vi "WLAN Tx Test Limits USL CarrierLeakage.vi"(8 "error in (no error)":errorcluster, 10 "Limits":T1 {"OBW"."Stop Frequency (Hz)" format="%#_4p"; "OBW"."Start Frequency (Hz)" format="%#_4p"; "OBW"."OBW (Hz)" format="%#_4p"}, 11 "WLAN Tx Test in":refnum<class "niDTS WLAN Tx Test.lvclass">) -> (0 "error out":errorcluster, 2 "Limits Out":T1 {"OBW"."Stop Frequency (Hz)" format="%#_4p"; "OBW"."Start Frequency (Hz)" format="%#_4p"; "OBW"."OBW (Hz)" format="%#_4p"}, 3 "WLAN Tx Test out":refnum<class "niDTS WLAN Tx Test.lvclass">)   [LabVIEW 2015, in "niDTS WLAN.lvlib" / "niDTS WLAN Tx Test.lvclass"]
uses:
  niDTS WLAN Tx Test.lvclass
  Includes/niDTS WLAN Tx Test INC Results.ctl
  Includes/niDTS WLAN Tx Test INC MOD EVM Results.ctl
  Includes/Results/niDTS Tx RES INC EVM.ctl
  Includes/niDTS WLAN Tx Test INC TXP Results.ctl
  Includes/niDTS WLAN Tx Test INC TXP Result SINGLE.ctl
  Includes/niDTS WLAN Tx Test INC OBW Results.ctl
  Instrument/INSTR TX/Results/niDTS WLAN INSTR TX INC SEM Results.ctl
  Instrument/INSTR TX/Results/niDTS WLAN INSTR TX INC SEM FSEGemts Results.ctl
  Includes/Results/niDTS Tx RES INC SEM FSEGemts.ctl
  Instrument/INSTR TX/Results/niDTS WLAN INSTR TX INC SEM MARGin Results.ctl
  Includes/Results/niDTS Tx RES INC SEM Margin.ctl
  Instrument/INSTR TX/Results/niDTS WLAN INSTR TX INC OFDM Impairments Results.ctl
  niDTS WLAN Tx Test.lvclass/niDTS WLAN Tx Test.ctl
  niDTS WLAN.lvlib
  Instrument/INSTR TX/niDTS WLAN INSTR TX.lvclass
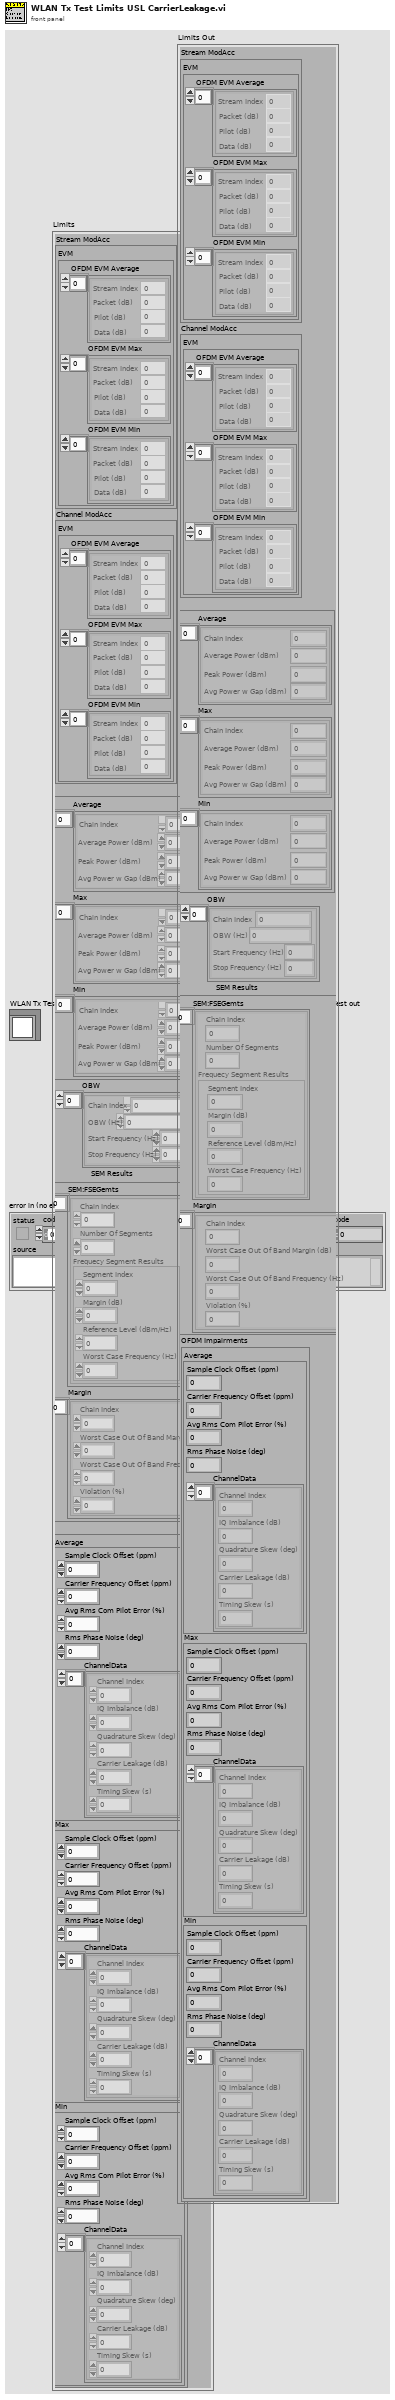
[diagram p1: front panel]
types:
  T1 = typedef "niDTS WLAN.lvlib/niDTS WLAN Tx Test INC Results.ctl" = cluster{"Stream ModAcc":T2, "Channel ModAcc":T2, "TXP":T4, "OBW":T6[], "SEM Results":T7, "OFDM Impairments":T12}
  T2 = typedef "niDTS WLAN.lvlib/niDTS WLAN Tx Test INC MOD EVM Results.ctl" = cluster{"EVM":cluster{"OFDM EVM Average":T3[], "OFDM EVM Max":T3[], "OFDM EVM Min":T3[]}}
  T3 = typedef "niDTS WLAN.lvlib/niDTS Tx RES INC EVM.ctl" = cluster{"Stream Index":i32, "Packet (dB)":dbl, "Pilot (dB)":dbl, "Data (dB)":dbl}
  T4 = typedef "niDTS WLAN.lvlib/niDTS WLAN Tx Test INC TXP Results.ctl" = cluster{"Average":T5[], "Max":T5[], "Min":T5[]}
  T5 = typedef "niDTS WLAN.lvlib/niDTS WLAN Tx Test INC TXP Result SINGLE.ctl" = cluster{"Chain Index":dbl, "Average Power (dBm)":dbl, "Peak Power (dBm)":dbl, "Avg Power w Gap (dBm)":dbl}
  T6 = typedef "niDTS WLAN.lvlib/niDTS WLAN Tx Test INC OBW Results.ctl" = cluster{"Chain Index":dbl, "OBW (Hz)":dbl, "Start Frequency (Hz)":dbl, "Stop Frequency (Hz)":dbl}
  T7 = typedef "niDTS WLAN.lvlib/niDTS WLAN INSTR TX.lvclass/niDTS WLAN INSTR TX INC SEM Results.ctl" = cluster{"SEM:FSEGemts":T8, "Margin":T10}
  T8 = typedef "niDTS WLAN.lvlib/niDTS WLAN INSTR TX.lvclass/niDTS WLAN INSTR TX INC SEM FSEGemts Results.ctl" = T9[]
  T9 = typedef "niDTS WLAN.lvlib/niDTS Tx RES INC SEM FSEGemts.ctl" = cluster{"Chain Index":i32, "Number Of Segments":i32, "Frequecy Segment Results":cluster{"Segment Index":i32, "Margin (dB)":dbl, "Reference Level (dBm/Hz)":dbl, "Worst Case Frequency (Hz)":dbl}}
  T10 = typedef "niDTS WLAN.lvlib/niDTS WLAN INSTR TX.lvclass/niDTS WLAN INSTR TX INC SEM MARGin Results.ctl" = T11[]
  T11 = typedef "niDTS WLAN.lvlib/niDTS Tx RES INC SEM Margin.ctl" = cluster{"Chain Index":i32, "Worst Case Out Of Band Margin (dB)":dbl, "Worst Case Out Of Band Frequency (Hz)":dbl, "Violation (%)":dbl}
  T12 = typedef "niDTS WLAN.lvlib/niDTS WLAN INSTR TX.lvclass/niDTS WLAN INSTR TX INC OFDM Impairments Results.ctl" = cluster{"Average":cluster{"Sample Clock Offset (ppm)":dbl, "Carrier Frequency Offset (ppm)":dbl, "Avg Rms Com Pilot Error (%)":dbl, "Rms Phase Noise (deg)":dbl, "ChannelData":cluster{"Channel Index":i32, "IQ Imbalance (dB)":dbl, "Quadrature Skew (deg)":dbl, "Carrier Leakage (dB)":dbl, "Timing Skew (s)":dbl}[]}, "Max":cluster{"Sample Clock Offset (ppm)":dbl, "Carrier Frequency Offset (ppm)":dbl, "Avg Rms Com Pilot Error (%)":dbl, "Rms Phase Noise (deg)":dbl, "ChannelData":cluster{"Channel Index":i32, "IQ Imbalance (dB)":dbl, "Quadrature Skew (deg)":dbl, "Carrier Leakage (dB)":dbl, "Timing Skew (s)":dbl}[]}, "Min":cluster{"Sample Clock Offset (ppm)":dbl, "Carrier Frequency Offset (ppm)":dbl, "Avg Rms Com Pilot Error (%)":dbl, "Rms Phase Noise (deg)":dbl, "ChannelData":cluster{"Channel Index":i32, "IQ Imbalance (dB)":dbl, "Quadrature Skew (deg)":dbl, "Carrier Leakage (dB)":dbl, "Timing Skew (s)":dbl}[]}}
  T13 = typedef "niDTS WLAN.lvlib/niDTS WLAN INC Standard.ctl" = enum16{"802.11 b DSSS", "802.11 a/g OFDM", "802.11 n HT", "802.11 ac VHT"}
  T14 = cluster{"Channel Index":i32, "IQ Imbalance (dB)":dbl, "Quadrature Skew (deg)":dbl, "Carrier Leakage (dB)":dbl, "Timing Skew (s)":dbl}[]
  T15 = cluster{"Channel Index":i32, "IQ Imbalance (dB)":dbl, "Quadrature Skew (deg)":dbl, "Carrier Leakage (dB)":dbl, "Timing Skew (s)":dbl}
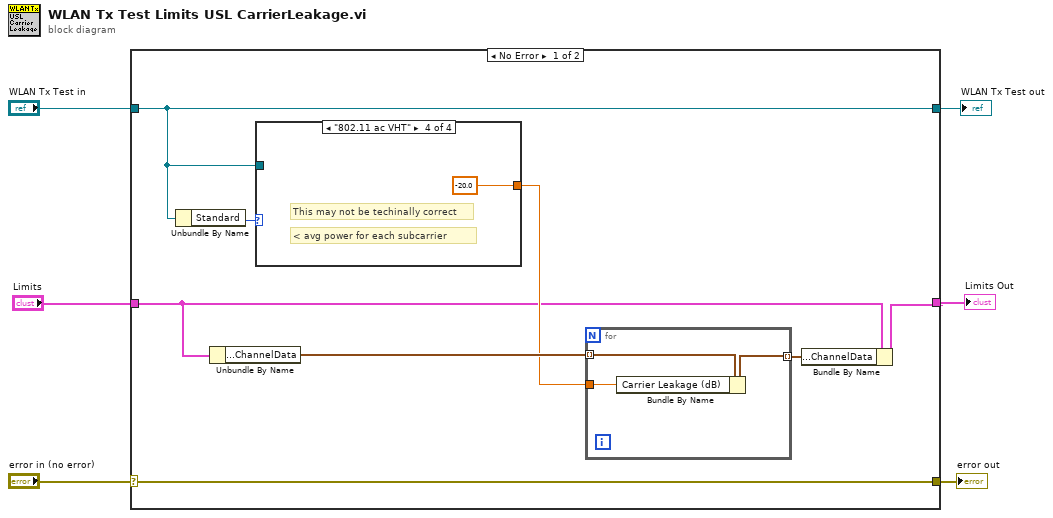
[diagram p0: block diagram]
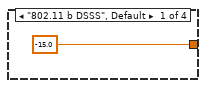
[diagram p2: hidden frame]
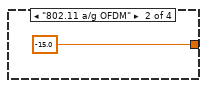
[diagram p3: hidden frame]
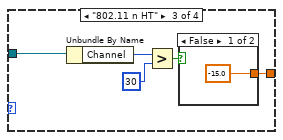
[diagram p4: hidden frame]
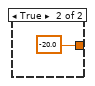
[diagram p5: hidden frame]
diagram:
  n1 = case shown="No Error" "error in (no error)" {
    selector: "error in (no error)" -> [w14 w30]
    tunnel: [w14 w30] -> w5
    tunnel: [w12 w29] -> w3
    tunnel: "WLAN Tx Test in" -> [w12 w29]
    tunnel: "Limits" -> [w9 w28]
    tunnel: [w7 w28] -> w1
    frame No Error {
      n2 = Unbundle By Name(w12) -> ("Standard"=w13:T13)
      n3 = Unbundle By Name(w9) -> ("OFDM Impairments.Average.ChannelData"=w11:T14)
      n4 = case shown="\"802.11 ac VHT\"" w13 {
        tunnel: w12 -> [_ _ w24 _]
        tunnel: [-15.0 -15.0 w20 -20.0] -> w10
        frame "802.11 b DSSS", Default {
        }
        frame "802.11 a/g OFDM" {
        }
        frame "802.11 n HT" {
          n5 = Unbundle By Name(w24) -> ("Channel"=w23:i32)
          n6 = Greater?(x=w23, y=30) -> (0:w21:bool)
          n7 = case shown="False" w21 {
            tunnel: [-15.0 -20.0] -> w20
            frame False {
            }
            frame True {
            }
          }
        }
        frame "802.11 ac VHT" {
          # "< avg power for each subcarrier"
          # "This may not be techinally correct"
        }
      }
      n8 = for {
        tunnel: w11 -> [w17] mode=indexing
        tunnel: [w16] -> w8 mode=indexing
        tunnel: w10 -> [w15]
        n9 = Bundle By Name(cluster=w17, "Carrier Leakage (dB)"=w15) -> (w16:T15)
      }
      n10 = Bundle By Name(cluster=w9, "OFDM Impairments.Average.ChannelData"=w8) -> (w7:T1)
    }
    frame Error {
    }
  }
  "error out" <- w5
  "WLAN Tx Test out" <- w3
  "Limits Out" <- w1
